vi "Q_Get Data for Flourish.vi"(8 "error in (no error)":errorcluster, 10 "Number of days":i32=7, 11 "Data Manager in":refnum<class "Data Manager.lvclass">) -> (0 "error out":errorcluster, 2 "Array":string[][](array[string]), 3 "Data Manager out":refnum<class "Data Manager.lvclass">)   [LabVIEW 2020, in "Data Manager.lvclass"]
uses:
  Data Manager.lvclass
  Data Manager.lvclass/Data Manager.ctl
  <vilib>/drjdpowell/SQLite Library/SQL Connection/Execute SQL (Single String).vi
  <vilib>/drjdpowell/SQLite Library/SQLite.lvlib
  <vilib>/addons/_JKI.lib/Serialization/JSON/Serializer/JSON Serializer/JSON Serializer.lvclass
  <vilib>/drjdpowell/SQLite Library/SQL Connection/Connection.lvclass
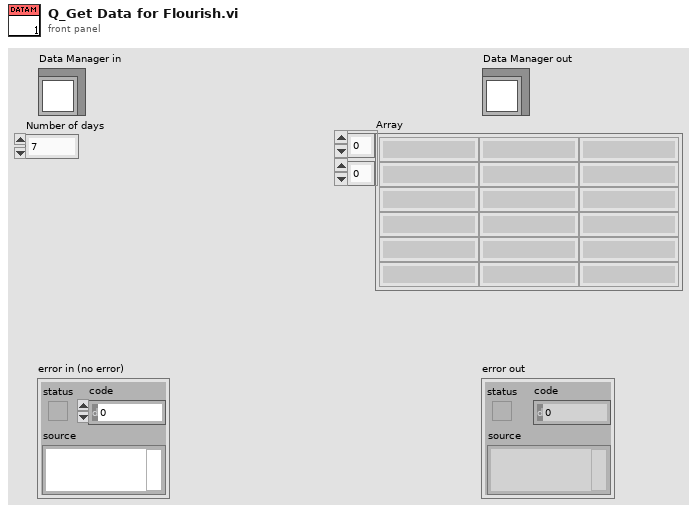
[diagram p1: front panel]
types:
  T1 = typedef "Data Manager.lvclass/Name--cluster.ctl" = cluster{"First":string, "Last":string}
  T2 = typedef "Data Manager.lvclass/Profile--cluster.ctl" = cluster{"Alias":string, "Team":string}
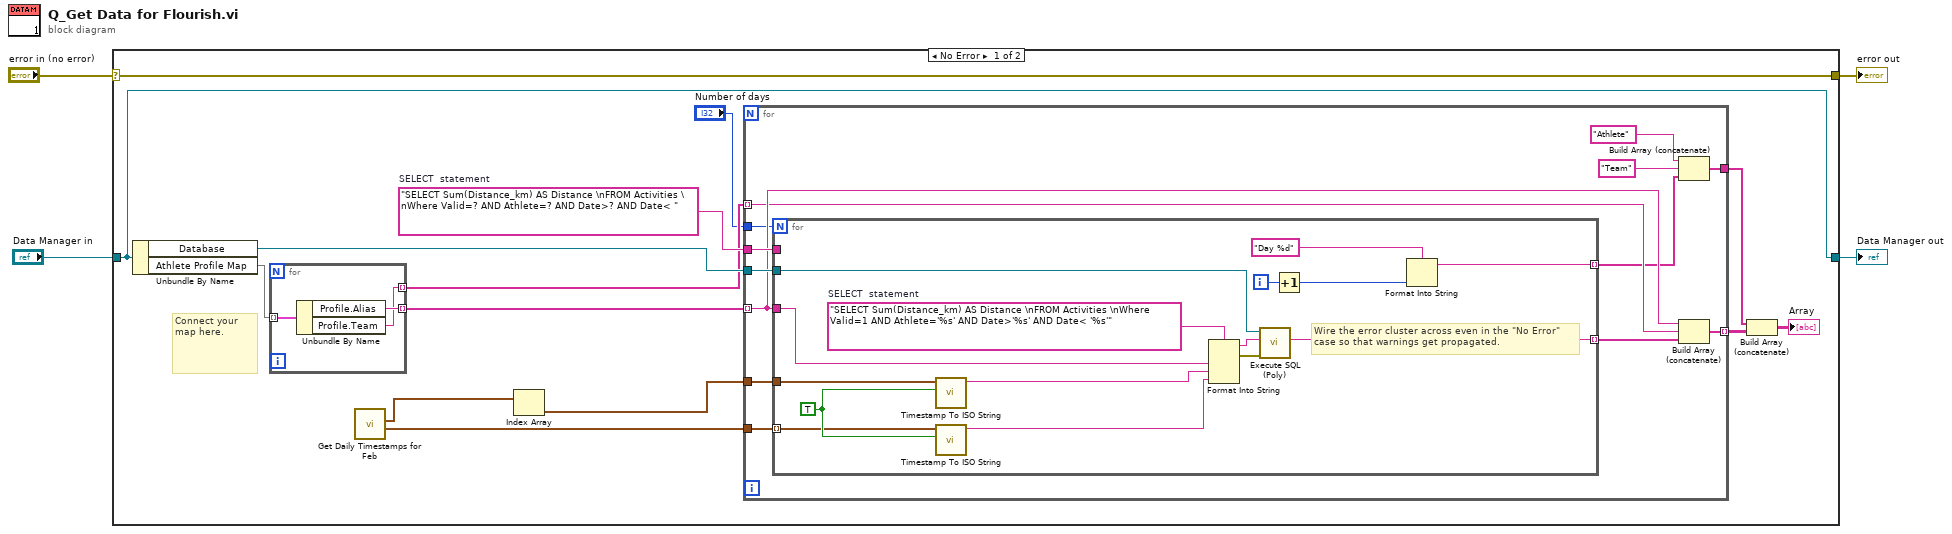
[diagram p0: block diagram]
diagram:
  n1 = case shown="No Error" "error in (no error)" {
    selector: "error in (no error)" -> [w18 w51]
    tunnel: [w18 w51] -> w3
    tunnel: [w16 w50] -> w1
    tunnel: "Data Manager in" -> [w16 w50]
    frame No Error {
      w17 = "SELECT Sum(Distance_km) AS Distance \nFROM Activities \nWhere Valid=? AND Athlete=? AND Date>? AND Date< "  # SELECT  statement
      # "Connect your map here."
      n2 = Unbundle By Name(w16) -> ("Database"=w15:refnum<class "Connection.lvclass">, "Athlete Profile Map"=w14:map{T1, T2})
      n3 = for {
        tunnel: w14 -> [w49] mode=indexing
        tunnel: [w48] -> w13 mode=indexing
        tunnel: [w47] -> w6 mode=indexing
        n4 = Unbundle By Name(w49) -> ("Profile.Alias"=w48:string, "Profile.Team"=w47:string)
      }
      n5 = call "Get Daily Timestamps for Feb.vi"() -> ("To"=w12:timestamp[], "From"=w11:timestamp[])  [unwired: 10 in]
      n6 = Index Array(array=w11) -> (element=w10:timestamp)  [unwired: 1 in]
      n7 = for {
        tunnel: w17 -> [w31]
        tunnel: w15 -> [w30]
        tunnel: w13 -> [w27] mode=indexing
        tunnel: w12 -> [w29]
        tunnel: w10 -> [w28]
        tunnel: [w25] -> w8 mode=indexing
        tunnel: [w22] -> w9
        tunnel: w6 -> [w24] mode=indexing
        tunnel: "Number of days" -> [w19]
        n8 = for {
          N: w19 -> [_]
          tunnel: w31 -> [_]
          tunnel: w30 -> [w46]
          tunnel: w27 -> [w37]
          tunnel: w28 -> [w43]
          tunnel: w29 -> [w39] mode=indexing
          tunnel: [w36] -> w26 mode=indexing
          tunnel: [w34] -> w23 mode=indexing
          i -> [w33]
          w42 = "SELECT Sum(Distance_km) AS Distance \nFROM Activities \nWhere Valid=1 AND Athlete='%s' AND Date>'%s' AND Date< '%s'"  # SELECT  statement
          w40 = TRUE ("Universal time (F)")
          # "Wire the error cluster across even in the \"No Error\"\ncase so that warnings get propagated."
          n9 = call <vilib>:"Timestamp To ISO String.vi"("Universal time (F)"=w40, "Timestamp"=w43) -> ("ISO Timestamp String"=w41:string)  [unwired: 8 in, 1 out]
          n10 = call <vilib>:"Timestamp To ISO String.vi"("Universal time (F)"=w40, "Timestamp"=w39) -> ("ISO Timestamp String"=w38:string)  [unwired: 8 in, 1 out]
          n11 = Format Into String(format string=w42, w37, w41, w38) -> (resulting string=w44:string, error out=w45:errorcluster)  [unwired: 2 in]
          n12 = call-poly <vilib>:"Execute SQL (Poly).vi"("error in (no error)"=w45, "SQL"=w44, "SQLite Connection in"=w46) -> ("Result"=w36:string)  [unwired: 6 in, 2 out]
          n13 = Increment(x=w33) -> (x+1=w32:i32)
          n14 = Format Into String(format string="Day %d", w32) -> (resulting string=w34:string)  [unwired: 2 in, 1 out]
        }
        n15 = Build Array (concatenate)("Athlete", "Team", w23) -> (w22:string[])
        n16 = Build Array (concatenate)(w27, w24, w26) -> (w25:string[])
      }
      n17 = Build Array (concatenate)(w9, w8) -> (→"Array":string[][])
    }
    frame Error {
    }
  }
  "error out" <- w3
  "Data Manager out" <- w1
